vi "LCP Get Flow Is.vi"(8 "error in (no error)":errorcluster caption="Fehler (Eingang, kein Fehler)", 11 "Pump Handle":i64) -> (0 "error out":errorcluster caption="Fehler (Ausgang)", 3 "Actual Flow Rate":dbl)   [LabVIEW 2023, in "labbCAN_Pump_API.lvlib"]
doc: "LCP_Func long LCP_CALL LCP_GetFlowIs(dev_hdl hPump, double *pFlowRateIs);"
uses:
  labbCAN_Pump_API.lvlib
  labbCAN_Pump_API.dll
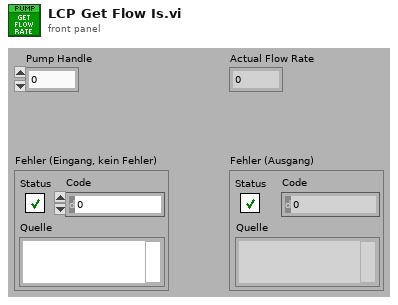
[diagram p1: front panel]
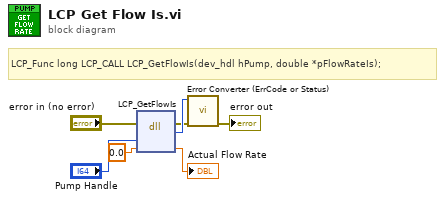
[diagram p0: block diagram]
diagram:
  # "LCP_Func long LCP_CALL LCP_GetFlowIs(dev_hdl hPump, double *pFlowRateIs);"
  n1 = dll-call lib="C:/GIT/AutomatedSetupAcousticEnergyDensity/CETONI_SDK/labbCAN_Pump_API.*" fn="LCP_GetFlowIs"(error in="error in (no error)", "hPump"="Pump Handle", "pFlowRateIs"=0.0) -> (error out=w2:errorcluster, "Rückgabetyp"=w3:i32, "pFlowRateIs"=→"Actual Flow Rate":dbl)  [unwired: 3 in, 1 out]
  n2 = call "Error Converter (ErrCode or Status).vi"("error in (no error)"=w2, "error code"=w3) -> ("error out"=→"error out":errorcluster)  [unwired: 9 in]
